vi "yolov9_openvino_video.vi"() -> ()   [LabVIEW 2018]
uses:
  <vilib>/addons/VIRobotics/ModelZoo/Object_Detection/yolov8_openvino/InitialModel_yolov9_OpenVINO_IR.vi
  <vilib>/addons/VIRobotics/opencv_yiku/Cap/Cap.lvclass
  <vilib>/addons/VIRobotics/ModelZoo/Object_Detection/yolov8_openvino/yolov8_openvino.lvclass
panel:
  in  "device_name":string(combo)="CPU"
  out "每帧耗时(s)":dbl
  in  "stop":bool
  out "picture":picture
  # "yolov9c OpenVINO 1280*720 on LabVIEW"
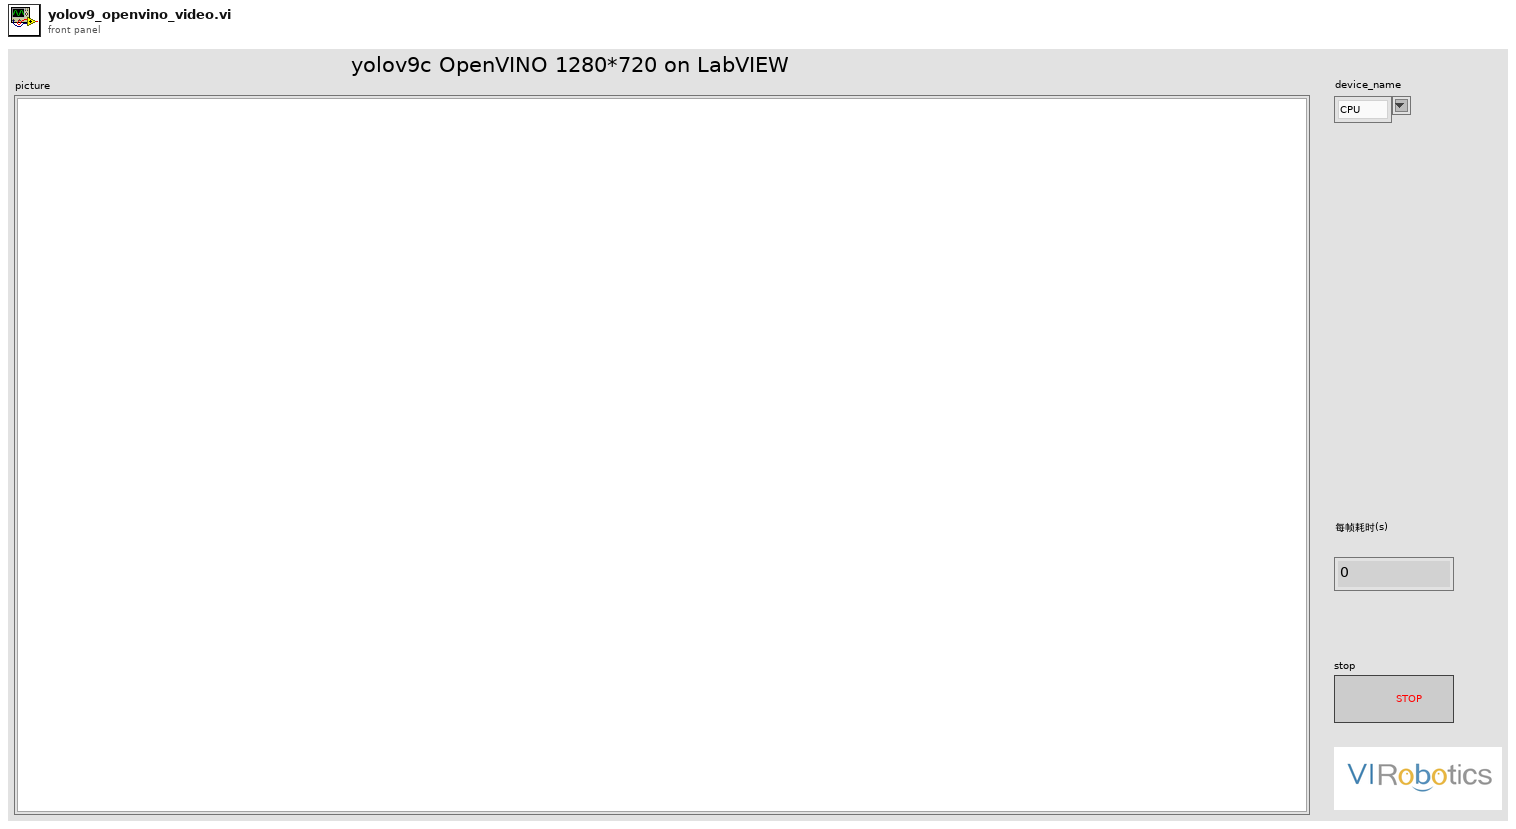
[diagram p1: front panel]
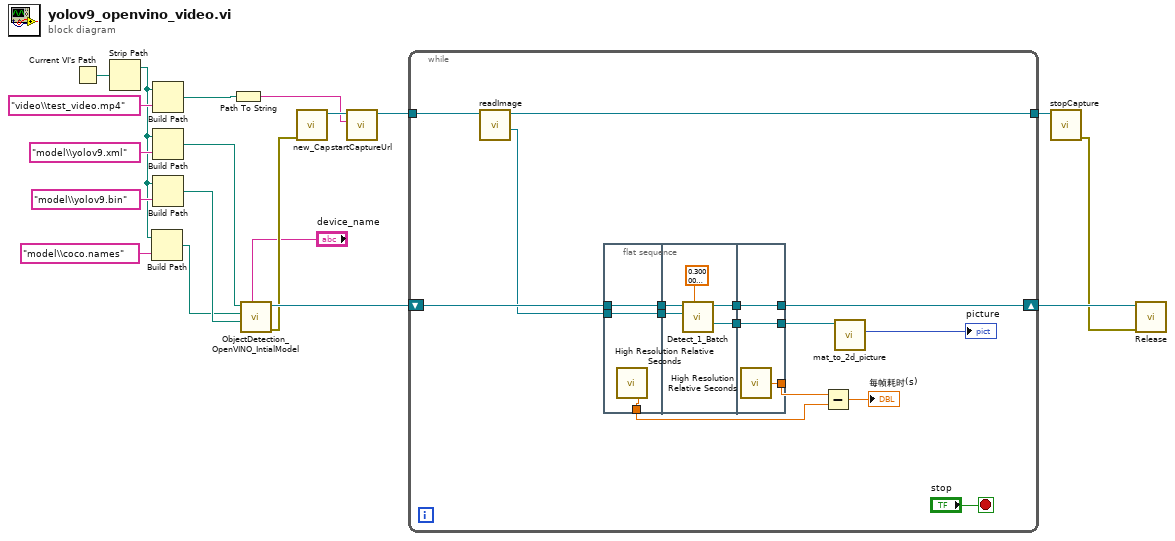
[diagram p0: block diagram]
diagram:
  n1 = Current VI's Path() -> (path=w9:path)
  n2 = Strip Path(path=w9) -> (stripped path=w1:path)  [unwired: 1 out]
  n3 = Build Path(base path=w1, name or relative path="model\\coco.names") -> (appended path=w2:path)
  n4 = Build Path(base path=w1, name or relative path="video\\test_video.mp4") -> (appended path=w10:path)
  n5 = Build Path(base path=w1, name or relative path="model\\yolov9.xml") -> (appended path=w5:path)
  n6 = Build Path(base path=w1, name or relative path="model\\yolov9.bin") -> (appended path=w4:path)
  n7 = Path To String(path=w10) -> (string=w14:string)
  n8 = call-poly <vilib>:"ObjectDetection_OpenVINO_IntialModel.vi"("device_name"="device_name", "bin_fle"=w4, "class_names_path"=w2, "xmlPath"=w5) -> ("error out"=w12:errorcluster, "yolov9_openvino out"=w13:refnum<class "yolov8_openvino.lvclass">)  [unwired: 6 in]
  n9 = call <vilib>:"new_Cap.vi"("error in (no error)"=w12) -> ("Cap out"=w16:refnum<class "Cap.lvclass">)  [unwired: 9 in, 1 out]
  n10 = call-dynamic "startCaptureUrl.vi"("url"=w14, "Cap in"=w16) -> ("Cap out"=w15:refnum<class "Cap.lvclass">)  [unwired: 8 in, 1 out]
  n11 = while {
    tunnel: w15 -> [w33]
    shift-right: [w30] -> w18
    shift-left: w13 -> [w34]
    tunnel: [w29] -> w19
    stop <- "stop" stop-if-true
    n12 = call <vilib>:"readImage.vi"("Cap in"=w33) -> ("Mat out"=w22:refnum<class "Mat_8U.lvclass">, "Cap out"=w29:refnum<class "Cap.lvclass">)  [unwired: 8 in, 1 out]
    n13 = flat-sequence {
      tunnel: w34 -> [w37]
      tunnel: [w37] -> w28
      tunnel: [w36] -> w24
      tunnel: w22 -> [w35]
      tunnel: [w35] -> w21
      tunnel: w28 -> [w42]
      tunnel: [w41] -> w27
      tunnel: [w40] -> w26
      tunnel: w21 -> [w39]
      tunnel: [w44] -> w30
      tunnel: [w45] -> w32
      tunnel: w27 -> [w45]
      tunnel: w26 -> [w44]
      tunnel: [w43] -> w25
      frame #0 {
        n14 = call <vilib>:"High Resolution Relative Seconds.vi"() -> ("relative seconds"=w36:dbl)
      }
      frame #1 {
        n15 = call-dynamic "Detect_1_Batch.vi"("confThreshold"=sgl 0.3, "image"=w39, "yolov8_openvino in"=w42) -> ("img out"=w41:refnum<class "Mat_8U.lvclass">, "yolov8_openvino out"=w40:refnum<class "yolov8_openvino.lvclass">)  [unwired: 5 in, 2 out]
      }
      frame #2 {
        n16 = call <vilib>:"High Resolution Relative Seconds.vi"() -> ("relative seconds"=w43:dbl)
      }
    }
    n17 = Subtract(x=w25, y=w24) -> (x-y=→"每帧耗时(s)":dbl)
    n18 = call <vilib>:"mat_to_2d_picture.vi"("Mat_8U in"=w32) -> ("picture"=→"picture":picture)  [unwired: 8 in, 2 out]
  }
  n19 = call <vilib>:"stopCapture.vi"("Cap in"=w19) -> ("error out"=w17:errorcluster)  [unwired: 10 in]
  n20 = call-dynamic "Release.vi"("error in (no error)"=w17, "yolov8_openvino in"=w18) -> ()  [unwired: 8 in, 2 out]
